vi "Get Server Address.vi"(11 "OOP Server in":refnum<class "MeasurementService_Template.lvclass">) -> (2 "Server Address":string, 3 "OOP Server out":refnum<class "MeasurementService_Template.lvclass">)   [LabVIEW 2020, in "MeasurementService_Template.lvlib" / "MeasurementService_Template.lvclass"]
uses:
  MeasurementService_Template.lvclass
  MeasurementService_Template.lvclass/MeasurementService_Template.ctl
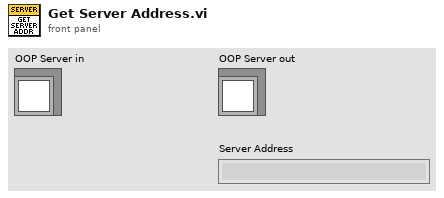
[diagram p1: front panel]
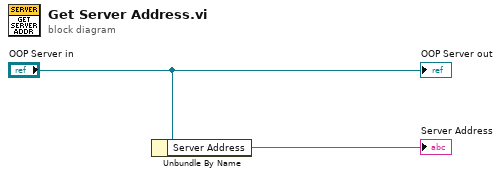
[diagram p0: block diagram]
diagram:
  n1 = Unbundle By Name("OOP Server in") -> ("Server Address"=→"Server Address":string)
  "OOP Server out" <- "OOP Server in"
